vi "VibrometerSettings.vi"(9 "OldVal":T1={"Name of test"="", "Date"=timestamp(0 s since 1904-01-01), "Location"="", "Template"="", "Soundcard"="", "resolution"=0, "Sampling rate"=0, "Ch1 Gain "=0.0, "Ch2 Gain"=0.0, "Sample time (s)"=0.0, "Pre-trigger (s)"=0.0, "Hammer Threshold"=0.0, "Positions"=0, "Taps/Position"=0, "Set Names"="", "Freq resolution"=0.0, "Hammer cutoff"=0.0, "Mic cutoff"=0.0, "Double bounce "=0.0, "Hammer Cal"=0.0, "dB Offset"=0.0, "Accel Cal"=0.0, "Vibrometer Cal"=0.0, "Mic Cal"=0.0, "Output"=0, "Voltage Cal"=0.0, "Vibrometer Port"="", "Range"=0, "High Pass"=0, "Bandwidth"=0, "X Range"=[], "Y Range"=[], "dB Spread"=0.0, "Trigger"=0, "Ch_1"=0, "Ch_2"=0, "flip?"=FALSE, "60Hz"=FALSE, "Time offset"=0.0, "Piezo Cal"=1.0, "Default Notes"="", "Tom"=FALSE} {"Ch_2" min=1 step=1; "Ch_1" min=1 max=100 step=1; "Trigger" items=["Hammer (force)", "Self-tap", "Spacebar"]; "Bandwidth" items=["1 kHz"=1, "5 kHz"=5, "10 kHz"=10, "25 kHz"=25, "50 kHz"=50, "100 kHz"=100]; "High Pass" items=["Off", "13 Hz", "104 Hz"]; "Range" items=["10 mm/s"=1, "20 mm/s"=2, "50 mm/s"=5, "100 mm/s"=10, "200 mm/s"=20, "500 mm/s"=50, "1 m/s"=100, "2 m/s"=200]; "Output" items=["Accelerometer", "Speed (from acceleration)", "Microphone", "Vibrometer", "Piezo"]; "Voltage Cal" format="%#_13g"; "Ch2 Gain" format="%#_13g"; "Ch1 Gain" format="%#_13g"; "Double bounce" min=0.0; "Mic cutoff" min=0.0 format="%#_4g"; "Hammer cutoff" min=0.0 format="%#_4g"; "Freq resolution" min=0.0; "Pre-trigger (s)" format="%#_13g"; "Date" format="%<%H:%M\n%d/%m/%y>T"; "resolution" items=["16 bit"=16, "24 bit"=24, "32 bit"=32]; "Sampling rate" items=["22050 samp/s"=22050, "44100 samp/s"=44100, "48000 samp/s"=48000]}, 11 "NewVal":T1={"Name of test"="", "Date"=timestamp(0 s since 1904-01-01), "Location"="", "Template"="", "Soundcard"="", "resolution"=0, "Sampling rate"=0, "Ch1 Gain "=0.0, "Ch2 Gain"=0.0, "Sample time (s)"=0.0, "Pre-trigger (s)"=0.0, "Hammer Threshold"=0.0, "Positions"=0, "Taps/Position"=0, "Set Names"="", "Freq resolution"=0.0, "Hammer cutoff"=0.0, "Mic cutoff"=0.0, "Double bounce "=0.0, "Hammer Cal"=0.0, "dB Offset"=0.0, "Accel Cal"=0.0, "Vibrometer Cal"=0.0, "Mic Cal"=0.0, "Output"=0, "Voltage Cal"=0.0, "Vibrometer Port"="", "Range"=0, "High Pass"=0, "Bandwidth"=0, "X Range"=[], "Y Range"=[], "dB Spread"=0.0, "Trigger"=0, "Ch_1"=0, "Ch_2"=0, "flip?"=FALSE, "60Hz"=FALSE, "Time offset"=0.0, "Piezo Cal"=1.0, "Default Notes"="", "Tom"=FALSE} {"Ch_2" min=1 step=1; "Ch_1" min=1 max=100 step=1; "Trigger" items=["Hammer (force)", "Self-tap", "Spacebar"]; "Bandwidth" items=["1 kHz"=1, "5 kHz"=5, "10 kHz"=10, "25 kHz"=25, "50 kHz"=50, "100 kHz"=100]; "High Pass" items=["Off", "13 Hz", "104 Hz"]; "Range" items=["10 mm/s"=1, "20 mm/s"=2, "50 mm/s"=5, "100 mm/s"=10, "200 mm/s"=20, "500 mm/s"=50, "1 m/s"=100, "2 m/s"=200]; "Output" items=["Accelerometer", "Speed (from acceleration)", "Microphone", "Vibrometer", "Piezo"]; "Voltage Cal" format="%#_13g"; "Ch2 Gain" format="%#_13g"; "Ch1 Gain" format="%#_13g"; "Double bounce" min=0.0; "Mic cutoff" min=0.0 format="%#_4g"; "Hammer cutoff" min=0.0 format="%#_4g"; "Freq resolution" min=0.0; "Pre-trigger (s)" format="%#_13g"; "Date" format="%<%H:%M\n%d/%m/%y>T"; "resolution" items=["16 bit"=16, "24 bit"=24, "32 bit"=32]; "Sampling rate" items=["22050 samp/s"=22050, "44100 samp/s"=44100, "48000 samp/s"=48000]}) -> (0 "Beam on":bool, 1 "update?":bool, 2 "Success?":bool, 3 "Settings":T1={"Name of test"="", "Date"=timestamp(0 s since 1904-01-01), "Location"="", "Template"="", "Soundcard"="", "resolution"=32, "Sampling rate"=48000, "Ch1 Gain "=25.0, "Ch2 Gain"=10.0, "Sample time (s)"=0.3, "Pre-trigger (s)"=0.01, "Hammer Threshold"=10.0, "Positions"=12, "Taps/Position"=5, "Set Names"="", "Freq resolution"=10.0, "Hammer cutoff"=0.0, "Mic cutoff"=0.0, "Double bounce "=0.0, "Hammer Cal"=1.0, "dB Offset"=0.0, "Accel Cal"=1.0, "Vibrometer Cal"=1.0, "Mic Cal"=1.0, "Output"=2, "Voltage Cal"=1.0, "Vibrometer Port"="ASRL27::INSTR", "Range"=50, "High Pass"=2, "Bandwidth"=25, "X Range"=[], "Y Range"=[], "dB Spread"=0.0, "Trigger"=0, "Ch_1"=1, "Ch_2"=2, "flip?"=FALSE, "60Hz"=FALSE, "Time offset"=0.0, "Piezo Cal"=1.0, "Default Notes"="", "Tom"=FALSE} {"Ch_2" min=1 step=1; "Ch_1" min=1 max=100 step=1; "Trigger" items=["Hammer (force)", "Self-tap", "Spacebar"]; "Bandwidth" items=["1 kHz"=1, "5 kHz"=5, "10 kHz"=10, "25 kHz"=25, "50 kHz"=50, "100 kHz"=100]; "High Pass" items=["Off", "13 Hz", "104 Hz"]; "Range" items=["10 mm/s"=1, "20 mm/s"=2, "50 mm/s"=5, "100 mm/s"=10, "200 mm/s"=20, "500 mm/s"=50, "1 m/s"=100, "2 m/s"=200]; "Output" items=["Accelerometer", "Speed (from acceleration)", "Microphone", "Vibrometer", "Piezo"]; "Voltage Cal" format="%#_13g"; "Ch2 Gain" format="%#_13g"; "Ch1 Gain" format="%#_13g"; "Double bounce" min=0.0; "Mic cutoff" min=0.0 format="%#_4g"; "Hammer cutoff" min=0.0 format="%#_4g"; "Freq resolution" min=0.0; "Pre-trigger (s)" format="%#_13g"; "Date" format="%<%H:%M\n%d/%m/%y>T"; "resolution" items=["16 bit"=16, "24 bit"=24, "32 bit"=32]; "Sampling rate" items=["22050 samp/s"=22050, "44100 samp/s"=44100, "48000 samp/s"=48000]}, 5 "update mic":bool)   [LabVIEW 2022 SP3]
uses:
  PreferencesControl.ctl
panel:
  # "Hz"
  # "dB"
  # "dB"
  # "sec"
  # "sec"
  # "mV/Pa"
  # "mV/m/s2"
  # "mV/mm/s"
  # "V/N"
  # "sec"
  # "sec"
  # "mV/N"
  # "a.u."
  # "a.u."
  # "sec"
  # "Hz"
  # "dB"
  # "dB"
  # "sec"
  # "sec"
  # "mV/Pa"
  # "mV/m/s2"
  # "mV/mm/s"
  # "V/N"
  # "sec"
  # "sec"
  # "mV/N"
  # "a.u."
  # "a.u."
  # "sec"
  # "Hz"
  # "dB"
  # "dB"
  # "sec"
  # "sec"
  # "mV/Pa"
  # "mV/m/s2"
  # "mV/mm/s"
  # "V/N"
  # "sec"
  # "sec"
  # "mV/N"
  # "a.u."
  # "a.u."
  # "sec"
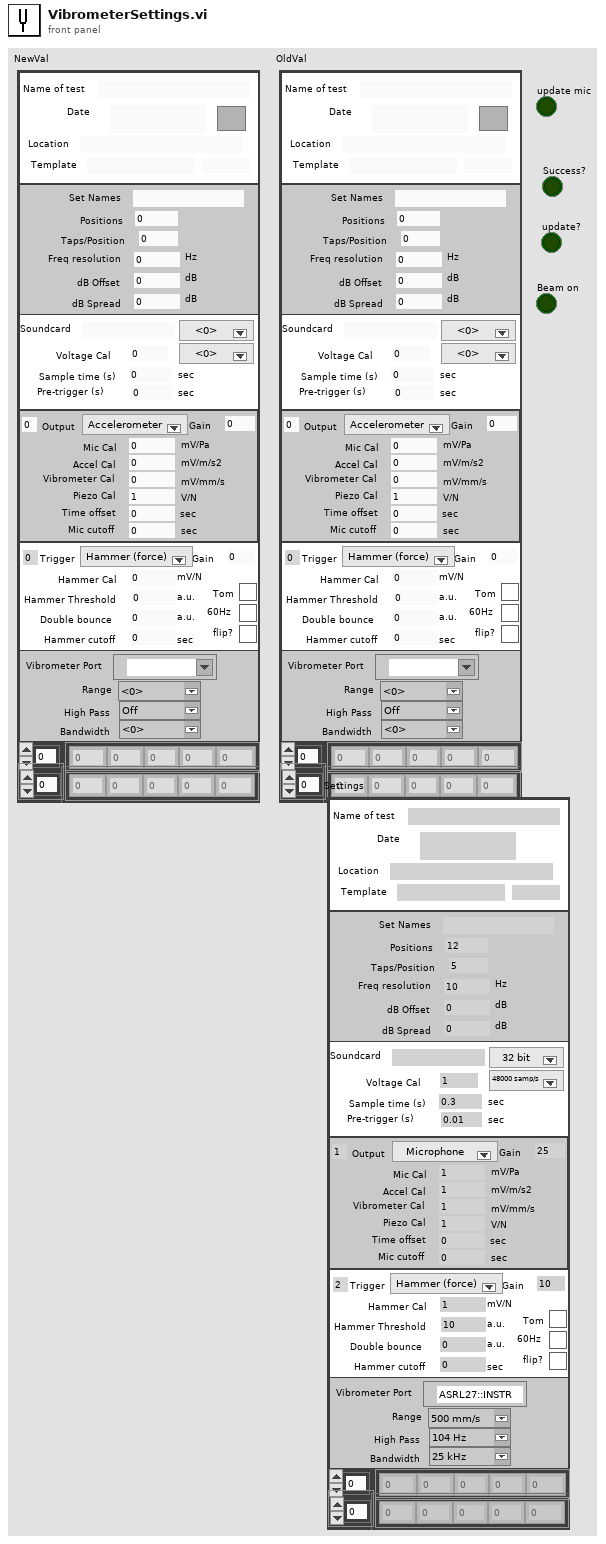
[diagram p1: front panel]
types:
  T1 = typedef "PreferencesControl.ctl" = cluster{"Name of test":string, "Date":timestamp, "Location":string, "Template":string, "Soundcard":string, "resolution":u16, "Sampling rate":u16, "Ch1 Gain ":dbl, "Ch2 Gain":dbl, "Sample time (s)":dbl, "Pre-trigger (s)":dbl, "Hammer Threshold":dbl, "Positions":i16, "Taps/Position":i16, "Set Names":string, "Freq resolution":dbl, "Hammer cutoff":dbl, "Mic cutoff":dbl, "Double bounce ":dbl, "Hammer Cal":dbl, "dB Offset":dbl, "Accel Cal":dbl, "Vibrometer Cal":dbl, "Mic Cal":dbl, "Output":u16, "Voltage Cal":dbl, "Vibrometer Port":refnum<visa-resource-name>, "Range":u16, "High Pass":u16, "Bandwidth":u16, "X Range":cluster{"Minimum":dbl, "Maximum":dbl, "Increment":dbl, "Minor Increment":dbl, "Start":dbl}[], "Y Range":cluster{"Minimum":dbl, "Maximum":dbl, "Increment":dbl, "Minor Increment":dbl, "Start":dbl}[], "dB Spread":dbl, "Trigger":u16, "Ch_1":u8, "Ch_2":u8, "flip?":bool, "60Hz":bool, "Time offset":dbl, "Piezo Cal":dbl, "Default Notes":string, "Tom":bool}
  T2 = cluster{"Name of test":bool, "Date":bool, "Location":bool, "Template":bool, "Soundcard":bool, "resolution":bool, "Sampling rate":bool, "Ch1 Gain ":bool, "Ch2 Gain":bool, "Sample time (s)":bool, "Pre-trigger (s)":bool, "Hammer Threshold":bool, "Positions":bool, "Taps/Position":bool, "Set Names":bool, "Freq resolution":bool, "Hammer cutoff":bool, "Mic cutoff":bool, "Double bounce ":bool, "Hammer Cal":bool, "dB Offset":bool, "Accel Cal":bool, "Vibrometer Cal":bool, "Mic Cal":bool, "Output":bool, "Voltage Cal":bool, "Vibrometer Port":bool, "Range":bool, "High Pass":bool, "Bandwidth":bool, "X Range":cluster{"Minimum":bool, "Maximum":bool, "Increment":bool, "Minor Increment":bool, "Start":bool}[], "Y Range":cluster{"Minimum":bool, "Maximum":bool, "Increment":bool, "Minor Increment":bool, "Start":bool}[], "dB Spread":bool, "Trigger":bool, "Ch_1":bool, "Ch_2":bool, "flip?":bool, "60Hz":bool, "Time offset":bool, "Piezo Cal":bool, "Default Notes":bool, "Tom":bool}
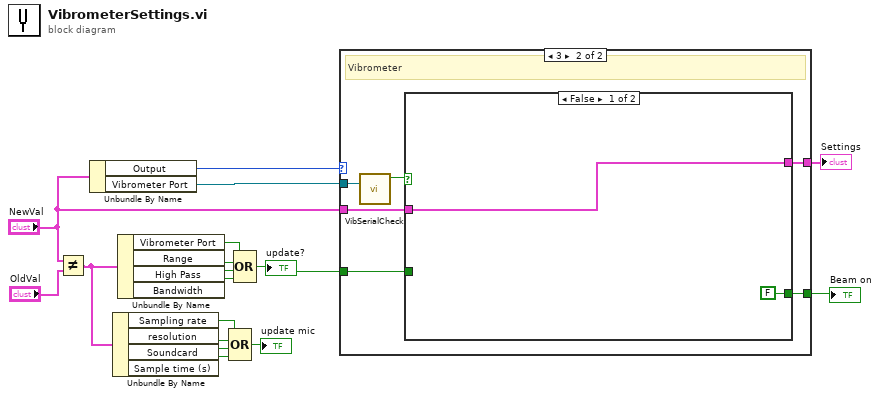
[diagram p0: block diagram]
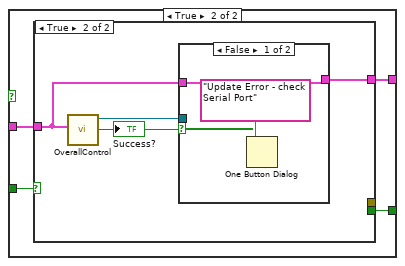
[diagram p3: hidden frame]
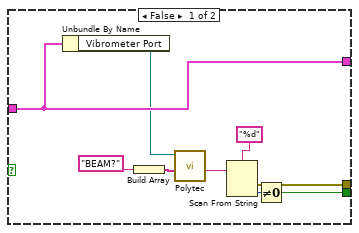
[diagram p4: hidden frame]
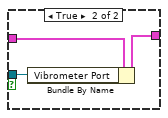
[diagram p5: hidden frame]
diagram:
  n1 = Not Equal?(x="NewVal", y="OldVal") -> (x != y?=w1:T2)
  n2 = Unbundle By Name("NewVal") -> ("Output"=w12:u16, "Vibrometer Port"=w7:refnum<visa-resource-name>)
  n3 = Unbundle By Name(w1) -> ("Sampling rate"=w2:bool, "resolution"=w3:bool, "Soundcard"=w4:bool, "Sample time (s)"=w5:bool)
  n4 = Unbundle By Name(w1) -> ("Vibrometer Port"=w16:bool, "Range"=w15:bool, "High Pass"=w14:bool, "Bandwidth"=w13:bool)
  n5 = Compound Arithmetic op=OR(w2, w3, w4, w5) -> (→"update mic":bool)
  n6 = Compound Arithmetic op=OR(w16, w15, w14, w13) -> (w10:bool)
  "update?" <- w10
  n7 = case shown="3" w12 {
    tunnel: "NewVal" -> [w18 w24]
    tunnel: w10 -> [_ w23]
    tunnel: [w18 w22] -> w9
    tunnel: [_ w21] -> w8
    tunnel: w7 -> [_ w20]
    frame 0, Default {
    }
    frame 3 {
      # "Vibrometer"
      n8 = call "VibSerialCheck.vi"("VISA Refnum in"=w20) -> ("Serial?"=w19:bool)  [unwired: 9 in, 1 out]
      n9 = case shown="False" w19 {
        tunnel: w24 -> [w26 w30]
        tunnel: w23 -> [_ w29]
        tunnel: [w26 w28] -> w22
        tunnel: [FALSE w27] -> w21
        frame False {
        }
        frame True {
          n10 = case shown="True" w29 {
            tunnel: w30 -> [w39 w42]
            tunnel: [w39 w40] -> w28
            tunnel: [w32 _] -> w27
            tunnel: [w31 _] -> _
            frame False {
              n11 = Unbundle By Name(w39) -> ("Vibrometer Port"=w38:refnum<visa-resource-name>)
              n12 = Build Array("BEAM?" ("format string")) -> (w36:string[])
              n13 = call "Polytec.vi"("RS232"=w38, "Strings"=w36) -> ("String Read"=w33:string)  [unwired: 7 in, 1 out]
              n14 = Scan From String(format string="%d", input string=w33) -> (error out=w31:errorcluster, output 1=w34:i32)  [unwired: 3 in, 2 out]
              n15 = Not Equal To 0?(x=w34) -> (x != 0?=w32:bool)
            }
            frame True {
              n16 = call "OverallControl.vi"("Settings"=w42) -> ("Success?"=w43:bool, "VISA Refnum out"=w41:refnum<visa-resource-name>)  [unwired: 9 in]
              "Success?" <- w43
              n17 = case shown="False" w43 {
                tunnel: w42 -> [w44 w48]
                tunnel: w41 -> [_ w47]
                tunnel: [w44 w46] -> w40
                frame False {
                  n18 = One Button Dialog(message="Update Error - check Serial Port") -> ()  [unwired: 1 in, 1 out]
                }
                frame True {
                  n19 = Bundle By Name(cluster=w48, "Vibrometer Port"=w47) -> (w46:T1)
                }
              }
            }
          }
        }
      }
    }
  }
  "Settings" <- w9
  "Beam on" <- w8
